vi "Data Types Exploration.vi"() -> ()   [LabVIEW 2026]
panel:
  out "String Output":string
  out "Integer 8 - OUTPUT":dbl
  in  "Integer 7 - INPUT":dbl
  out "String Output":string
  out "Integer 6 - OUTPUT":dbl
  in  "Integer 5 - INPUT":dbl
  out "Floating Point Nmber 3 - OUTPUT":dbl
  out "Integer 4 - OUTPUT":i32
  in  "Integer 3 - INPUT":i32
  out "String Output":string
  in  "String Input":string
  out "Boolean 2":bool
  in  "Boolean":bool
  out "Integer 2 - Output":i32
  in  "Integer 1 - Input":i32
  out "Float Point Numeric 2":dbl
  in  "Float Point Numeric 1":dbl
  # "Understanding Data Types"
  # "Understanding Compatible Data type Conversion (Int to Float)"
  # "Visualising Incompatible Type (Broken Wire)"
  # "Visualising String to Integer converter"
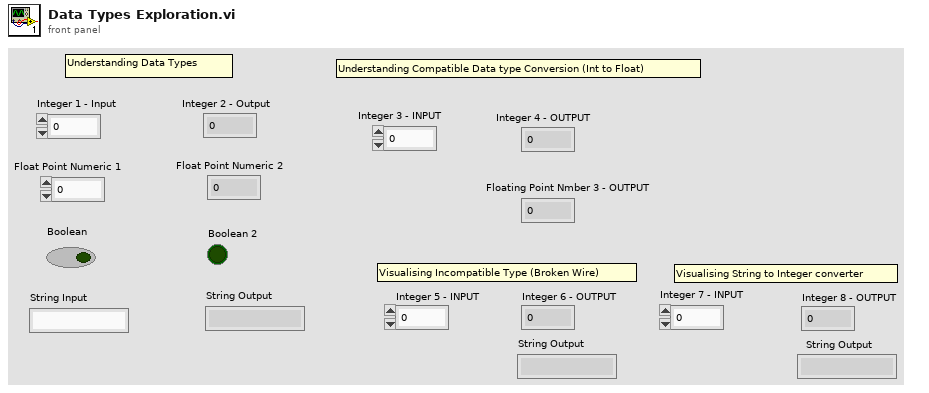
[diagram p1: front panel]
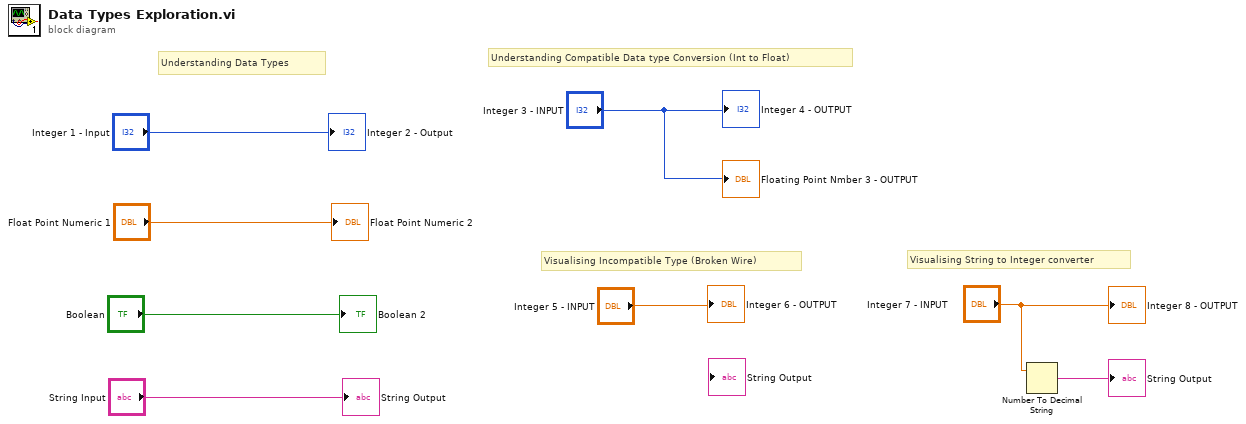
[diagram p0: block diagram]
diagram:
  # "Visualising String to Integer converter"
  # "Visualising Incompatible Type (Broken Wire)"
  # "Understanding Compatible Data type Conversion (Int to Float)"
  # "Understanding Data Types"
  n1 = Number To Decimal String(number="Integer 7 - INPUT") -> (decimal integer string=→"String Output":string)  [unwired: 1 in]
  "Float Point Numeric 2" <- "Float Point Numeric 1"
  "Integer 2 - Output" <- "Integer 1 - Input"
  "Boolean 2" <- "Boolean"
  "String Output" <- "String Input"
  "Integer 4 - OUTPUT" <- "Integer 3 - INPUT"
  "Floating Point Nmber 3 - OUTPUT" <- "Integer 3 - INPUT"
  "Integer 6 - OUTPUT" <- "Integer 5 - INPUT"
  "Integer 8 - OUTPUT" <- "Integer 7 - INPUT"
